vi "VI, Set Pane Origin.vi"(4 "y (0)":i16, 5 "x (0)":i16, 6 "error in":errorcluster, 8 "index (0)":i32, 9 "VI ref":refnum<vi>) -> (0 "error out":errorcluster, 3 "VI ref dup":refnum<vi>)   [LabVIEW 2010]
doc: "This function sets the origin (vertical and horizontal coordinates of the upper left corner of the pane) for one pane in a panel. Changing the origin enables scrolling the pane. The coordinates are relative to the coordinate system of the pane."
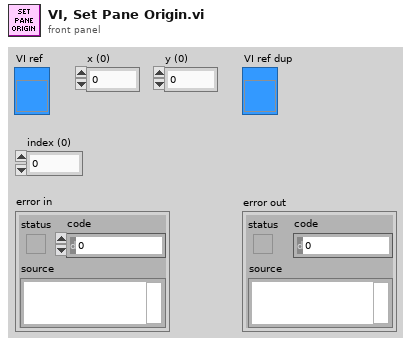
[diagram p1: front panel]
types:
  T1 = typedef "LVPointTypeDef.ctl" = cluster{"Horizontal":i16, "Vertical":i16}
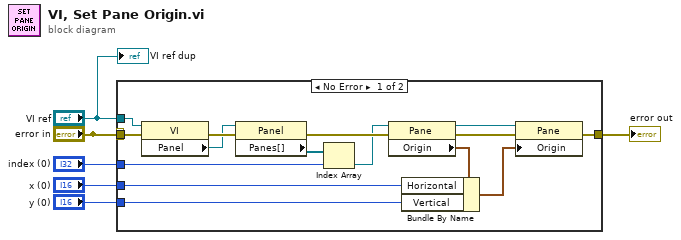
[diagram p0: block diagram]
diagram:
  n1 = case shown="No Error" "error in" {
    selector: "error in" -> [_ w22]
    tunnel: [w17 w22] -> w6
    tunnel: "VI ref" -> [w20 _]
    tunnel: "error in" -> [w21 _]
    tunnel: "x (0)" -> [w10 _]
    tunnel: "y (0)" -> [w9 _]
    tunnel: "index (0)" -> [w11 _]
    frame No Error {
      n2 = property class="VI"(reference=w20, error in=w21) -> (error out=w19:errorcluster, "Panel"=w18:refnum<vi>)  [unwired: 1 out]
      n3 = property class="Panel"(reference=w18, error in=w19) -> (error out=w15:errorcluster, "Panes[]"=w16:refnum<vi>[])  [unwired: 1 out]
      n4 = Index Array(array=w16, index=w11) -> (element=w8:refnum<vi>)
      n5 = property class="Pane"(reference=w8, error in=w15) -> (reference out=w7:refnum<vi>, error out=w14:errorcluster, "Origin"=w13:T1)
      n6 = Bundle By Name(cluster=w13, "Horizontal"=w10, "Vertical"=w9) -> (w12:T1)
      n7 = property class="Pane"(reference=w7, error in=w14, "Origin"=w12) -> (error out=w17:errorcluster)  [unwired: 1 out]
    }
    frame Error {
    }
  }
  "error out" <- w6
  "VI ref dup" <- "VI ref"
